vi "NMRvmeCard6.vi"() -> ()   [LabVIEW 2013]
uses:
  <vilib>/Utility/file.llb/Read From Spreadsheet File (DBL).vi
  <vilib>/Analysis/NI_AALBase.lvlib
panel:
  out "Diff Sigma":dbl=0.0021417004437574343 format="%#_13g"
  out "Peak center (MHz)":sgl=213.00386 format="%.3f"
  out "Peak width (MHz)":sgl=0.03243152 format="%.5f"
  in  "Max":bool
  in  "Logoffset (V)":dbl=-5.996000000000003 min=-9.0 max=0.0 step=0.0005 format="%_5g"
  in  "Phase (V)":dbl=6.500000000000002 min=0.0 max=9.0 step=0.0005 format="%_5g"
  out "Telnet error out":errorcluster
  in  "Real/Quad Q curve":bool=TRUE
  out "Temperature (C)":dbl(graph)=26.25
  out "+3V supply":dbl=3.245 format="%_4g"
  out "Temp (C)":dbl=26.25 format="%_4g"
  in  "RemovePed":bool=TRUE
  in  "IF / LOG Det":bool
  in  "Q curve file":string="realback212a.txt"
  out "File name 2":string="C:\\users\\plm\\Desktop\\rssmt\\realback212a.txt"
  in  "AutoTune":bool
  out "RF OK":bool=TRUE
  out "Peak area (V-MHz)":sgl=0.0028527237 format="%.5f"
  in  "Gauss Fit":bool
  out "NMR Graph + Fit":cluster{cluster{dbl, "Numeric":dbl}[]}[](graph)=[{[{212.6, "Numeric"=-0.001303666666666866}, {212.60999999999999, "Numeric"=-0.0012636666666681479}, {212.62, "Numeric"=-0.00035966666666543273}, {212.63, "Numeric"=-0.0006916666666666911}, {212.64, "Numeric"=-0.00025966666666788624}, {212.65, "Numeric"=-0.0006636666666653777}, {212.66, "Numeric"=-0.00020366666666654307}, {212.67, "Numeric"=0.00012033333333236022}, {212.68, "Numeric"=-0.0002916666666653491}, {212.69, "Numeric"=0.001060333333333583}, {212.7, "Numeric"=0.0009763333333325762}, {212.71, "Numeric"=0.0011563333333346557}, {212.72, "Numeric"=0.0010003333333336792}, {212.73, "Numeric"=0.0015083333333327717}, {212.74, "Numeric"=0.001480333333331924}, {212.75, "Numeric"=0.0017163333333337534}, {212.76, "Numeric"=0.0018163333333329357}, {212.77, "Numeric"=0.0019803333333321847}, {212.78, "Numeric"=0.0016083333333338007}, {212.79, "Numeric"=0.001300333333333079}, {212.8, "Numeric"=0.0008563333333324215}, {212.81, "Numeric"=0.00037633333333382535}, {212.82, "Numeric"=0.000660333333333196}, {212.82999999999998, "Numeric"=0.0012083333333326321}, {212.84, "Numeric"=0.001520333333333822}, {212.85, "Numeric"=0.001796333333333287}, {212.85999999999999, "Numeric"=0.0017363333333328176}, {212.87, "Numeric"=0.0022403333333337943}, {212.88, "Numeric"=0.0025083333333333537}, {212.89, "Numeric"=0.0023403333333329775}, {212.9, "Numeric"=0.003036333333333742}, {212.91, "Numeric"=0.0030963333333333953}, {212.92, "Numeric"=0.002320333333333113}, {212.93, "Numeric"=0.002808333333333664}, {212.94, "Numeric"=0.005660333333333411}, {212.95, "Numeric"=0.006976333333333223}, {212.96, "Numeric"=0.00985633333333356}, {212.97, "Numeric"=0.019200333333333403}, {212.98, "Numeric"=0.034408333333333305}, {212.99, "Numeric"=0.03538033333333328}, {213.0, "Numeric"=0.02571633333333337}, {213.01, "Numeric"=0.021516333333333366}, {213.02, "Numeric"=0.020180333333333432}, {213.03, "Numeric"=0.015108333333333307}, {213.04, "Numeric"=0.014500333333333401}, {213.05, "Numeric"=0.014356333333333561}, {213.06, "Numeric"=0.012676333333333224}, {213.07, "Numeric"=0.015160333333333411}, {213.08, "Numeric"=0.011308333333333663}, {213.09, "Numeric"=0.006820333333333113}, {213.1, "Numeric"=0.003896333333333395}, {213.11, "Numeric"=0.002636333333333742}, {213.12, "Numeric"=0.0027403333333329786}, {213.13, "Numeric"=0.0011083333333333535}, {213.14000000000001, "Numeric"=4.033333333379463e-05}, {213.15, "Numeric"=-0.0013636666666671828}, {213.16, "Numeric"=0.0001963333333332871}, {213.17000000000002, "Numeric"=0.0005203333333338219}, {213.18, "Numeric"=0.002208333333332632}, {213.19, "Numeric"=0.0014603333333331955}, {213.2, "Numeric"=0.0009763333333338252}, {213.21, "Numeric"=0.00035633333333242104}, {213.22, "Numeric"=-0.0006996666666669211}, {213.23, "Numeric"=-0.0023916666666661986}, {213.24, "Numeric"=-0.0017196666666654085}, {213.25, "Numeric"=-0.0012836666666670646}, {213.26, "Numeric"=-0.0025836666666662466}, {213.27, "Numeric"=-0.002919666666665363}, {213.28, "Numeric"=-0.0018916666666672285}, {213.29, "Numeric"=-0.0006996666666663209}, {213.3, "Numeric"=-0.0006436666666653455}, {213.31, "Numeric"=-0.0012236666666674244}, {213.32, "Numeric"=-0.0005396666666664159}, {213.33, "Numeric"=-9.166666666534859e-05}, {213.34, "Numeric"=-0.0004796666666676396}, {213.35, "Numeric"=-3.6666666665425424e-06}, {213.36, "Numeric"=-0.0009636666666653776}, {213.37, "Numeric"=-0.00025966666666788624}, {213.38, "Numeric"=-0.0004916666666666923}, {213.39000000000001, "Numeric"=0.0004403333333345659}, {213.4, "Numeric"=-0.0008636666666681468}]}]
  in  "Amp of Q curve":dbl=1.8000000000000034 min=0.0 max=29.0 step=0.01 format="%_3f"
  in  "Subtract Q curve":bool=TRUE
  out "Pedestal Offset":dbl(graph)=-0.007420833333333359
  out "Pedestal Difference":dbl(graph)=-0.001148999999999757
  out "# Good Spectra":i32=1
  in  "Quality cuts":bool=TRUE
  out "Pedestal OK":bool=TRUE
  out "Sweep #":i32=70
  out "1st Sweep":bool
  out "ADC volts OK":bool=TRUE
  out "Peak Height Distribution":cluster{"Y":dbl[], "Y":dbl[]}[](graph)=[{"Y"=[0.03253033333333327, 0.03253033333333327, 0.03253033333333327, 0.03253033333333327, 0.03253033333333327, 0.03253033333333327, 0.03253033333333327, 0.03253033333333327, 0.03253033333333327, 0.03253033333333327, 0.03253033333333327, 0.03253033333333327, 0.03253033333333327, 0.03253033333333327, 0.03253033333333327, 0.03253033333333327, 0.03253033333333327, 0.03253033333333327, 0.03253033333333327, 0.03253033333333327, 0.03253033333333327, 0.03253033333333327, 0.03253033333333327, 0.03253033333333327, 0.03253033333333327, 0.03253033333333327, 0.03253033333333327, 0.03253033333333327, 0.03253033333333327, 0.03253033333333327, 0.03253033333333327, 0.03253033333333327, 0.03253033333333327, 0.03253033333333327, 0.03253033333333327, 0.03253033333333327, 0.03253033333333327, 0.03253033333333327, 0.03253033333333327, 0.03253033333333327, 0.03253033333333327, 0.03253033333333327, 0.03253033333333327, 0.03253033333333327, 0.03253033333333327, 0.03253033333333327, 0.03253033333333327, 0.03253033333333327, 0.03253033333333327, 0.03253033333333327, 0.03253033333333327, 0.03253033333333327, 0.03253033333333327, 0.03253033333333327, 0.03253033333333327, 0.03253033333333327, 0.03253033333333327, 0.03253033333333327, 0.03253033333333327, 0.03253033333333327, 0.03253033333333327, 0.03253033333333327, 0.03253033333333327, 0.03253033333333327, 0.03253033333333327, 0.03253033333333327, 0.03253033333333327, 0.03253033333333327, 0.03253033333333327, 0.03253033333333327, 0.03253033333333327, 0.03253033333333327, 0.03253033333333327, 0.03253033333333327, 0.03253033333333327, 0.03253033333333327, 0.03253033333333327, 0.03253033333333327, 0.03253033333333327, 0.03253033333333327, 0.03253033333333327, 0.03253033333333327, 0.03253033333333327, 0.03253033333333327, 0.03253033333333327, 0.03253033333333327, 0.03253033333333327, 0.03253033333333327, 0.03253033333333327, 0.03253033333333327, 0.03253033333333327, 0.03253033333333327, 0.03253033333333327, 0.03253033333333327, 0.03253033333333327, 0.03253033333333327, 0.03253033333333327, 0.03253033333333327, 0.03253033333333327, 0.03253033333333327], "Y"=[0.0, 0.0, 0.0, 0.0, 0.0, 0.0, 0.0, 0.0, 0.0, 0.0, 0.0, 0.0, 0.0, 0.0, 0.0, 0.0, 0.0, 0.0, 0.0, 0.0, 0.0, 0.0, 0.0, 0.0, 0.0, 0.0, 0.0, 0.0, 0.0, 0.0, 0.0, 0.0, 0.0, 0.0, 0.0, 0.0, 0.0, 0.0, 0.0, 0.0, 0.0, 0.0, 0.0, 0.0, 0.0, 0.0, 0.0, 0.0, 0.0, 0.0, 0.0, 0.0, 0.0, 0.0, 0.0, 0.0, 0.0, 0.0, 0.0, 0.0, 0.0, 0.0, 0.0, 0.0, 0.0, 0.0, 0.0, 0.0, 0.0, 0.0, 0.0, 0.0, 0.0, 0.0, 0.0, 0.0, 0.0, 0.0, 0.0, 0.0, 0.0, 0.0, 0.0, 0.0, 0.0, 0.0, 0.0, 0.0, 0.0, 0.0, 0.0, 0.0, 0.0, 0.0, 0.0, 0.0, 0.0, 0.0, 0.0, 1.0]}]
  in  "# of Sweeps":i32=1000
  out "S/N":dbl=nan format="%_3g"
  out "Peak mean (V)":dbl=0.03253033333333327 format="%_4g"
  out "Peak Height":dbl(graph)=0.03538033333333328
  in  "Raw Data":bool=TRUE
  in  "Tank RF":bool=TRUE
  in  "IF Atten (dB)":i8=3 min=0 max=31 step=1
  in  "IFoffset (V)":dbl=5.366811000000014 min=-0.0 max=9.0 step=0.001 format="%.4f"
  in  "Tune  (V)":dbl=0.34700000000000086 min=-0.5 max=8.0 step=0.001 format="%.4f"
  in  "Hi / Lo Gain":bool
  out "Voltage Array":sgl[](array[numeric])=[0.0208, 0.0194, 0.0189, 0.0172, 0.0163, 0.0146, 0.0138, 0.0129, 0.0113, 0.0115, 0.0103, 0.0094, 0.0082, 0.0077, 0.0067, 0.006, 0.0052, 0.0045, 0.0033, 0.0022, 0.001, -0.0002, -0.0006, -0.0007, -0.001, -0.0013, -0.0019, -0.0019, -0.0021, -0.0027, -0.0024, -0.0027, -0.0038, -0.0036, -0.001, 0.0001, 0.0028, 0.012, 0.0271, 0.028, 0.0183, 0.0141, 0.0128, 0.0078, 0.0073, 0.0073, 0.0058, 0.0085, 0.0049, 0.0007, -0.0019, -0.0028, -0.0023, -0.0035, -0.0041, -0.005, -0.0029, -0.002, 0.0003, 0.0002, 0.0004, 0.0005, 0.0002, -0.0007, 0.0008, 0.0021, 0.0017, 0.0023, 0.0043, 0.0065, 0.0076, 0.0081, 0.0099, 0.0115, 0.0123, 0.014, 0.0143, 0.0163, 0.0174, 0.0197, 0.0198] format="%.4f"
  in  "Invert Polarity":bool=TRUE
  out "Pedestal Diff (V)":sgl=-0.001149 format="%.3f"
  out "Peak amp (V)":sgl=0.035380334 format="%.3f"
  in  "Save Data to File":bool
  in  "RF Level (dBm)":dbl min=-10.0 max=10.0 step=0.1 format="%.2f"
  out "SMT error out":errorcluster
  out "Sample RMS (V)":dbl=0.0007950617283950617 format="%.4f"
  in  "# Sample/step":i32=70 min=1 max=5000 step=100
  in  "Step Width (MHz)":dbl=0.01 min=0.0 max=1000.0 step=0.0001 format="%.4f"
  in  "Freq Span (MHz)":dbl=0.8 min=0.0 max=3000.0 step=0.1 format="%.3f"
  in  "Center Freq (MHz)":dbl=213.0 min=0.005 max=6000.0 step=0.1 format="%.3f"
  in  "Sweep Mode":u16(ring)=3 items=["Off", "Single", "Auto", "Step"]
  in  "GPIB Addr (28)":refnum<visa-resource-name>="GPIB0::28::INSTR"
  # "E1039 Prototype NMR Control Panel"
  # "Settings"
  # "D\nA\nC"
  # "R\nF\n\nG\nE\nN \n\n+\n\nI\nF"
  # "A\nD\nC"
  # "I\n/\nO"
  # "D\nA\nT\nA\n\nA \nN\nA\nL\nY\nS\nI\nS"
  # "Results"
  # "A\nv\ne\nr\na\ng\ne"
  # "S\nw\ne\ne\np"
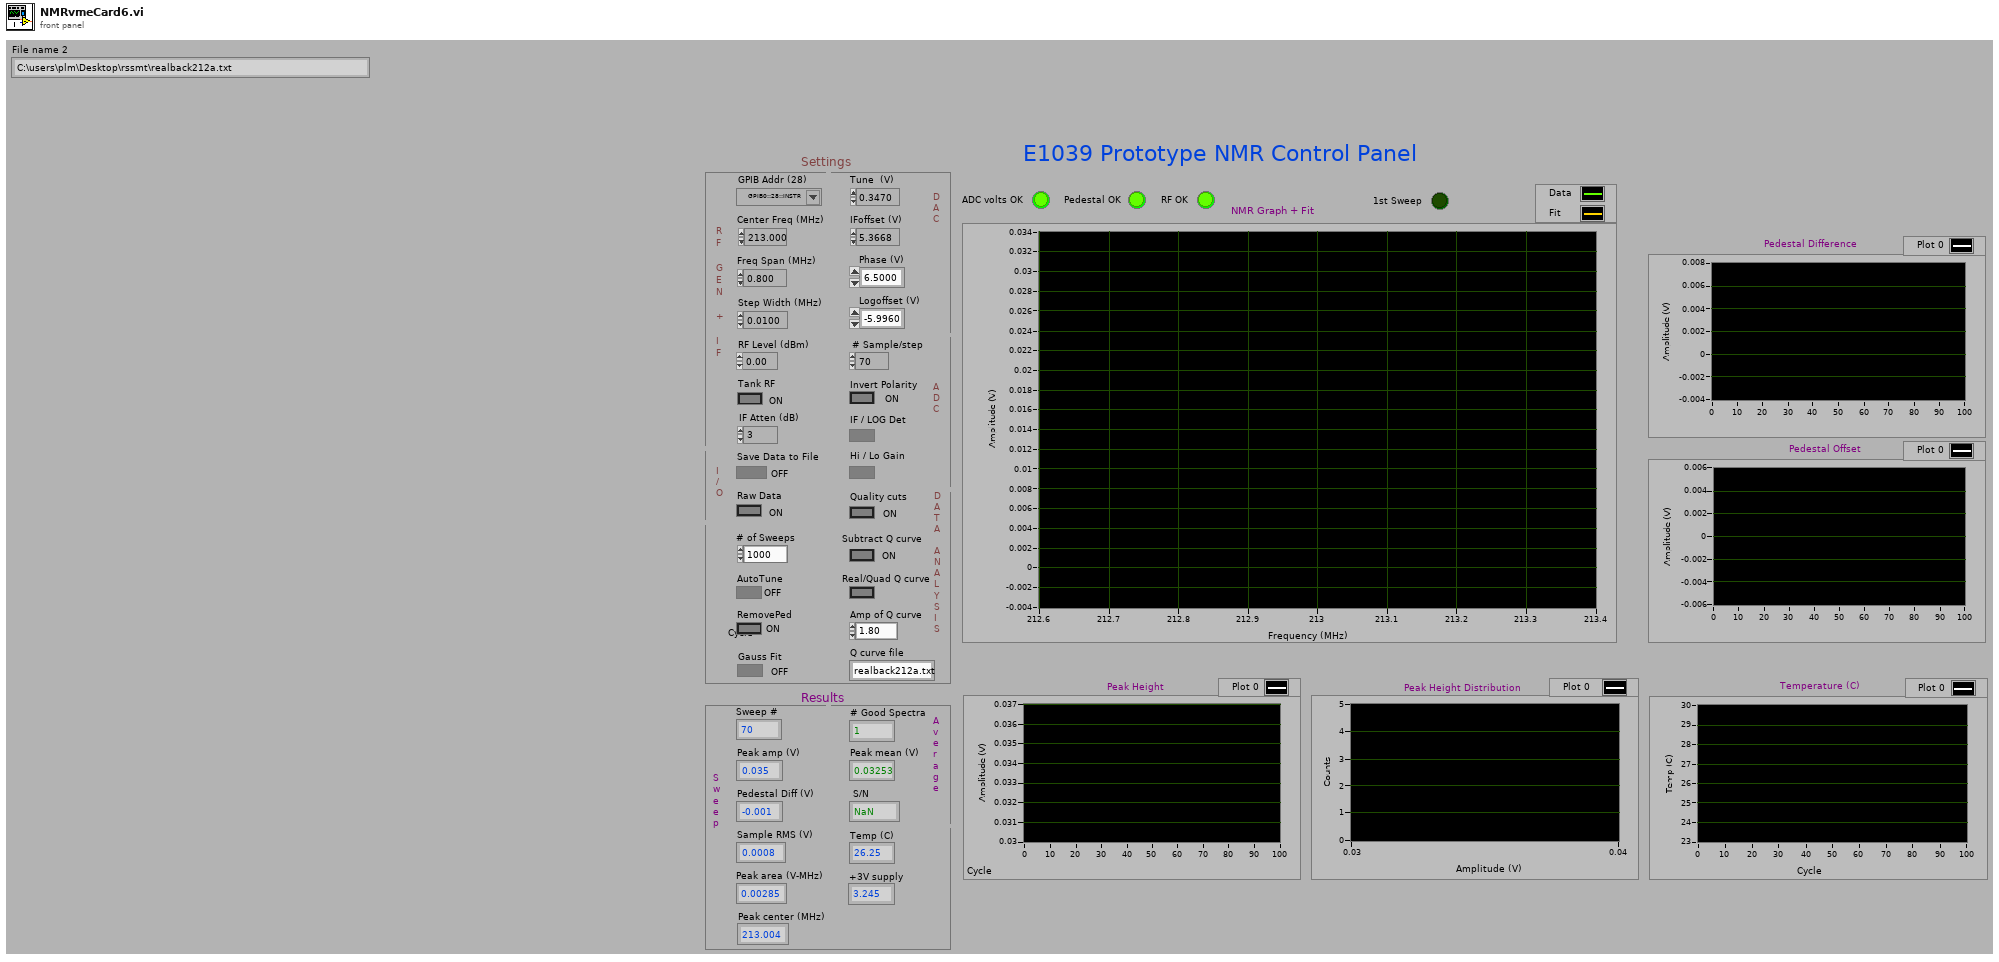
[diagram p1: front panel]
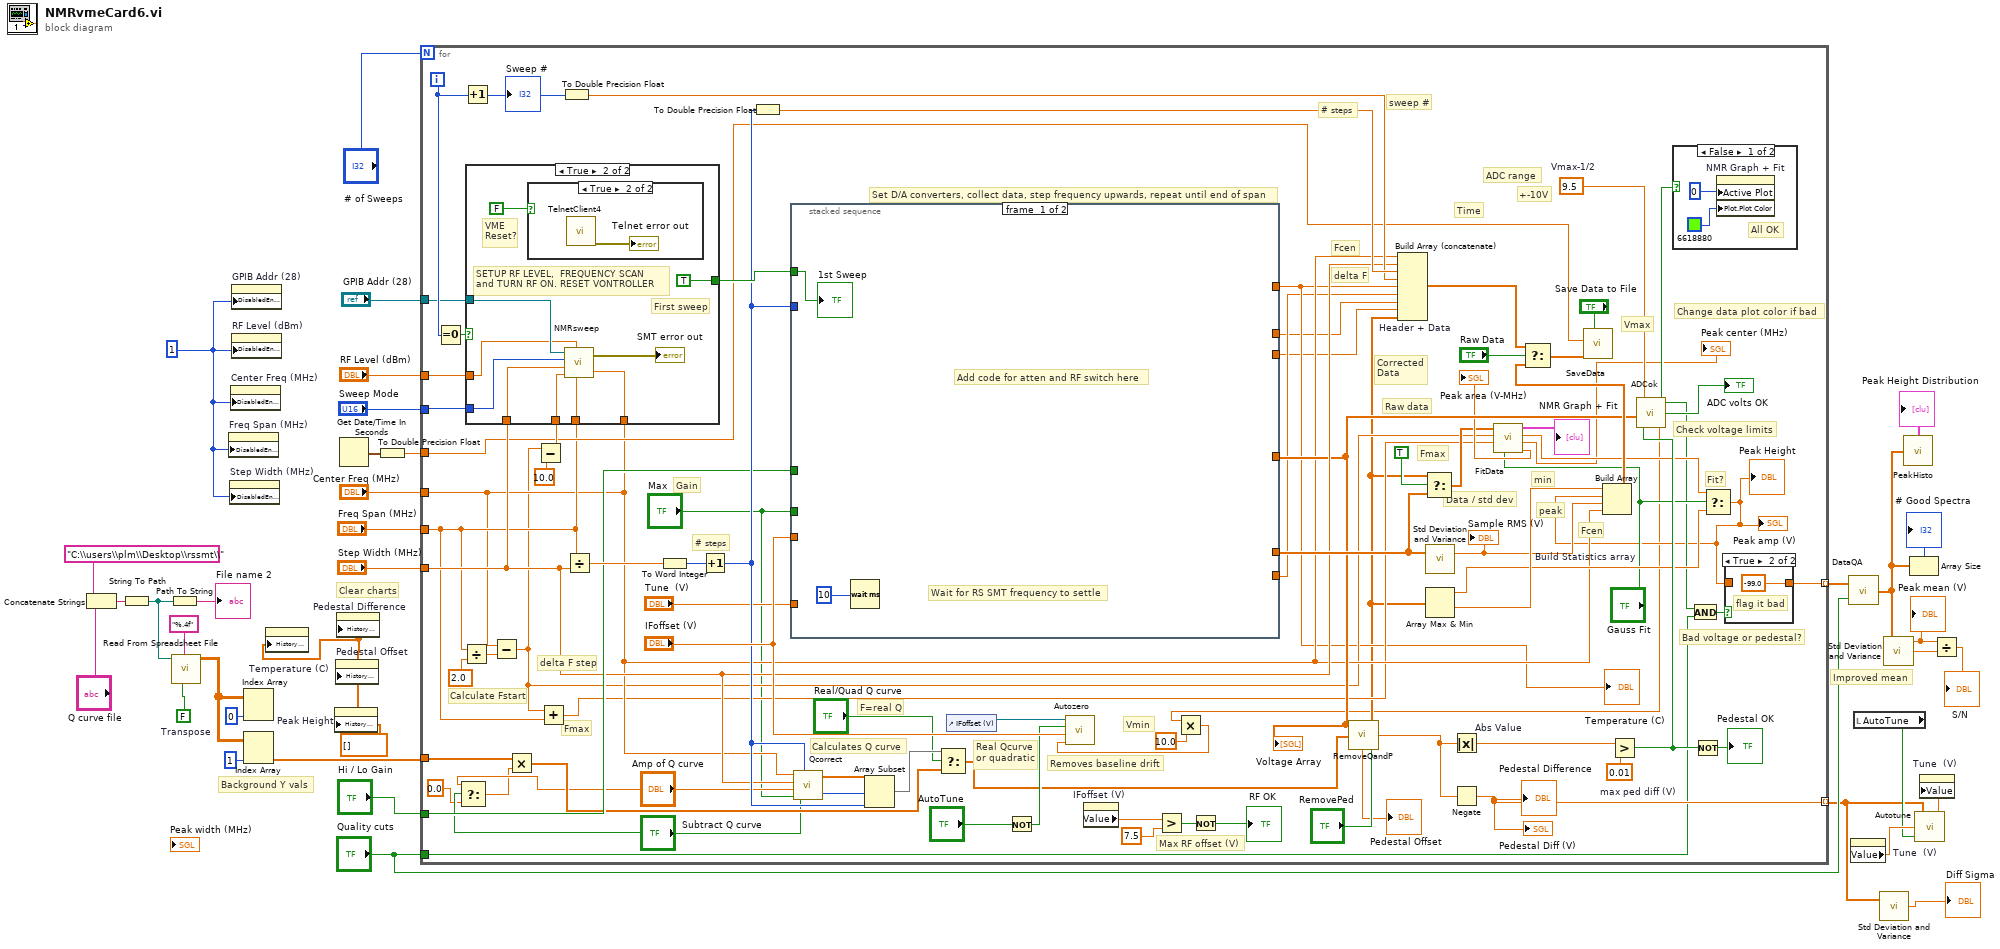
[diagram p0: block diagram]
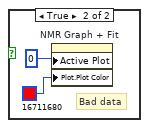
[diagram p2: hidden frame]
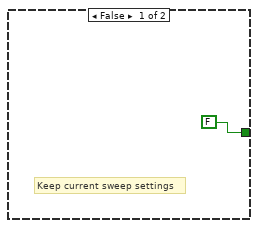
[diagram p4: hidden frame]
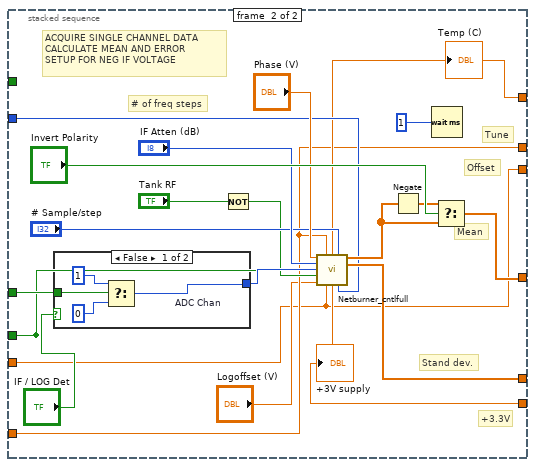
[diagram p6: hidden frame]
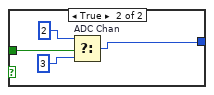
[diagram p7: hidden frame]
diagram:
  w4 = 1
  w16 = FALSE  # Transpose
  w8 = dbl[] []
  # "Background Y vals"
  # "Clear charts"
  # "Improved mean"
  n1 = Concatenate Strings "Concatenate Strings"("C:\\users\\plm\\Desktop\\rssmt\\", "Q curve file") -> (w19:string)
  n2 = String To Path(string=w19) -> (path=w15:path)
  n3 = Path To String(path=w15) -> (string=→"File name 2":string)
  n4 = call-poly <vilib>:"Read From Spreadsheet File.vi"("transpose (no:F)"=w16, "format (%.3f)"="%.4f", "file path (dialog if empty)"=w15) -> ("all rows"=w14:dbl[][])  [unwired: 4 in, 4 out]
  n5 = property on="Freq Span (MHz)" class="DigNum (strict)"("DisabledEnum"=w4) -> ()  [unwired: 2 in, 2 out]
  n6 = property on="Step Width (MHz)" class="DigNum (strict)"("DisabledEnum"=w4) -> ()  [unwired: 2 in, 2 out]
  n7 = property on="Center Freq (MHz)" class="DigNum (strict)"("DisabledEnum"=w4) -> ()  [unwired: 2 in, 2 out]
  n8 = property on="GPIB Addr (28)" class="VISAName"("DisabledEnum"=w4) -> ()  [unwired: 2 in, 2 out]
  n9 = property on="RF Level (dBm)" class="DigNum (strict)"("DisabledEnum"=w4) -> ()  [unwired: 2 in, 2 out]
  n10 = Index Array "Index Array"(array=w14, index (col)=0) -> ()  [unwired: 1 in, 1 out]
  n11 = Index Array(array=w14, index (col)=1) -> (element=w9:dbl[])  [unwired: 1 in]
  n12 = property on="Temperature (C)" class="WFChart (strict)"("History Data"=w8) -> ()  [unwired: 2 in, 2 out]
  n13 = property on="Peak Height" class="WFChart (strict)"("History Data"=w8) -> ()  [unwired: 2 in, 2 out]
  n14 = property on="Pedestal Offset" class="WFChart (strict)"("History Data"=w8) -> ()  [unwired: 2 in, 2 out]
  n15 = property on="Pedestal Difference" class="WFChart (strict)"("History Data"=w8) -> ()  [unwired: 2 in, 2 out]
  n16 = Get Date/Time In Seconds() -> (seconds since 1Jan1904=w21:timestamp)
  n17 = To Double Precision Float(number=w21) -> (double precision float=w20:dbl)
  n18 = for {
    N: "# of Sweeps" -> [_]
    tunnel: [w104] -> w34 mode=indexing
    tunnel: "Quality cuts" -> [w83]
    tunnel: [w88] -> w2 mode=indexing
    tunnel: "Center Freq (MHz)" -> [w70]
    tunnel: "Freq Span (MHz)" -> [w76]
    tunnel: "Step Width (MHz)" -> [w82]
    tunnel: "Sweep Mode" -> [w92]
    tunnel: "Hi / Lo Gain" -> [w91]
    tunnel: "GPIB Addr (28)" -> [w90]
    tunnel: "RF Level (dBm)" -> [w89]
    tunnel: w20 -> [w77]
    tunnel: w9 -> [w55]
    i -> [w102]
    w86 = 9.5  # Vmax-1/2
    w105 = 0.01  # max ped diff (V)
    # "Gain"
    # "F=real Q"
    # "Real Qcurve\nor quadratic"
    # "+-10V"
    # "Vmax"
    # "Change data plot color if bad"
    # "Max RF offset (V)"
    # "Fmax"
    # "Fit?"
    # "Fmax"
    # "Time"
    # "Vmin"
    # "min"
    # "peak"
    # "Raw data"
    # "Corrected\nData"
    # "Fcen"
    # "delta F"
    # "# steps"
    # "ADC range"
    # "sweep #"
    # "Fcen"
    # "Set D/A converters, collect data, step frequency upwards, repeat until end of span"
    # "Calculates Q curve"
    # "Removes baseline drift"
    # "Bad voltage or pedestal?"
    # "Check voltage limits"
    # "Data / std dev"
    # "# steps"
    # "Calculate Fstart"
    # "delta F step"
    n19 = Equal To 0?(x=w102) -> (x = 0?=w107:bool)
    n20 = Select(t="Amp of Q curve", s="Subtract Q curve", f=0.0) -> (s? t:f=w50:dbl)
    n21 = Divide(x=w76, y=sgl 2.0) -> (x/y=w118:dbl)
    n22 = Increment(x=w102) -> (x+1=w93:i32)
    "Sweep #" <- w93
    n23 = Subtract(x=w70, y=w118) -> (x-y=w65:dbl)
    n24 = Multiply(x=w55, y=w50) -> (x*y=w54:dbl[])
    n25 = Subtract(x=w65, y=10.0) -> (x-y=w116:dbl)
    n26 = case shown="True" w107 {
      tunnel: w116 -> [_ w137]
      tunnel: w82 -> [_ w135]
      tunnel: w70 -> [_ w134]
      tunnel: w76 -> [_ w136]
      tunnel: [FALSE TRUE] -> w106
      tunnel: w92 -> [_ w131]
      tunnel: w90 -> [_ w130]
      tunnel: w89 -> [_ w129]
      frame False {
        # "Keep current sweep settings"
      }
      frame True {
        # "VME\nReset?"
        # "First sweep"
        # "SETUP RF LEVEL,  FREQUENCY SCAN\nand TURN RF ON. RESET VONTROLLER"
        n27 = case shown="True" FALSE {
          frame False {
          }
          frame True {
            n28 = call "TelnetClient4.vi"() -> ("Telnet error"=→"Telnet error out":errorcluster)  [unwired: 4 in, 3 out]
          }
        }
        n29 = call "NMRsweep.vi"("Center Freq (MHz)"=w134, "Freq Span (MHz)"=w136, "RF Level (dBm)"=w129, "Foffset (MHz)"=w137, "Step Width (MHz)"=w135, "Sweep Mode"=w131, "GPIB Addr (28)"=w130) -> ("error out"=→"SMT error out":errorcluster)
      }
    }
    n30 = Add(x=w65, y=w76) -> (x+y=w64:dbl)
    n31 = To Double Precision Float(number=w93) -> (double precision float=w94:dbl)
    n32 = Divide(x=w76, y=w82) -> (x/y=w120:dbl)
    n33 = To Word Integer(number=w120) -> (16bit integer=w117:i16)
    n34 = Increment(x=w117) -> (x+1=w96:i16)
    n35 = To Double Precision Float(number=w96) -> (double precision float=w95:dbl)
    n36 = stacked-sequence {
      tunnel: [_ w152] -> w110
      tunnel: [_ w159] -> w80
      tunnel: w96 -> [_ w149]
      tunnel: "IFoffset (V)" -> [_ w142]
      tunnel: w91 -> [_ w157]
      tunnel: w106 -> [w139 _]
      tunnel: "Tune  (V)" -> [_ w144]
      tunnel: [_ w148] -> w46
      tunnel: [_ w145] -> w45
      tunnel: [_ w144] -> w43
      tunnel: [_ w142] -> w42
      tunnel: [_ w141] -> _
      tunnel: "Max" -> [_ w141]
      frame #0 {
        # "Add code for atten and RF switch here"
        # "Wait for RS SMT frequency to settle"
        n37 = Wait (ms)(milliseconds to wait=10) -> ()  [unwired: 1 out]
        "1st Sweep" <- w139
      }
      frame #1 {
        # "+3.3V"
        # "Offset"
        # "Tune"
        # "Stand dev."
        # "Mean"
        # "ACQUIRE SINGLE CHANNEL DATA\nCALCULATE MEAN AND ERROR\nSETUP FOR NEG IF VOLTAGE"
        # "# of freq steps"
        n38 = case shown="False" "IF / LOG Det" {
          tunnel: w157 -> [w165 w166]
          tunnel: [w162 w167] -> w151
          frame False {
            n39 = Select "ADC Chan"(t=1, s=w165, f=0) -> (s? t:f=w162:i32)
          }
          frame True {
            n40 = Select "ADC Chan"(t=2, s=w166, f=3) -> (s? t:f=w167:i32)
          }
        }
        n41 = Not(x="Tank RF") -> (.not. x?=w147:bool)
        n42 = call "Netburner_cntlfull.vi"("Phase Volt"="Phase (V)", "Tune Volt"=w144, "# Data"="# Sample/step", "IF Atten (dB)"="IF Atten (dB)", "NMR ADC"=w151, "Hi Gain"=w141, "Tank RF"=w147, "LogOff Volt"="Logoffset (V)", "IFOff Volt"=w142, "# f steps"=w149) -> ("Temp (C)"=w148:dbl, "ADC value"=w153:dbl[], "ADC error"=w152:dbl[], "Volts"=w145:dbl)  [unwired: 2 out]
        "Temp (C)" <- w148
        "+3V supply" <- w145
        n43 = Negate(x=w153) -> (-x=w158:dbl[])
        n44 = Wait (ms)(milliseconds to wait=1) -> ()  [unwired: 1 out]
        n45 = Select(t=w158, s="Invert Polarity", f=w153) -> (s? t:f=w159:dbl[])
      }
    }
    "Voltage Array" <- w80
    "Temperature (C)" <- w46
    n46 = call "Qcorrect.vi"("Subtract Q curve"="Subtract Q curve", "Nstep"=w96, "Max Gain"="Max", "Amp of Q curve"="Amp of Q curve", "Step Width (MHz)"=w82, "Center Freq (MHz)"=w70) -> ("Start"=w111:i32, "Array"=w112:dbl[])
    n47 = Array Subset "Array Subset"(array=w112, index=w111, length=w96) -> (w58:dbl[])
    n48 = Select(t=w58, s="Real/Quad Q curve", f=w54) -> (s? t:f=w57:dbl[])
    n49 = control-ref of="IFoffset (V)"() -> (w85:refnum<vi>)
    n50 = Not(x="AutoTune") -> (.not. x?=w59:bool)
    n51 = property on="IFoffset (V)" class="DigNum (strict)"() -> ("Value"=w74:dbl)  [unwired: 2 in, 2 out]
    n52 = Greater?(x=w74, y=7.5) -> (0:w72:bool)
    n53 = Not(x=w72) -> (.not. x?=→"RF OK":bool)
    n54 = call "RemoveQandP.vi"("Subtract Ped?"="RemovePed", "Qcurve"=w57, "Raw data"=w80) -> ("Ped L-R"=w98:dbl, "Corrected data"=w44:dbl[], "Ped Offfset"=→"Pedestal Offset":dbl)
    n55 = Build Array (concatenate) "Header + Data"(w70, w82, w95, w94, w46, w45, w43, w42, w44) -> (w97:dbl[])
    n56 = Select(t=w44, s=TRUE, f=w110) -> (s? t:f=w66:dbl[])
    n57 = call <vilib>:"Std Deviation and Variance.vi"("X"=w110) -> ("mean"=w81:dbl)  [unwired: 1 in, 2 out]
    "Sample RMS (V)" <- w81
    n58 = Array Max & Min(array=w44) -> (max value=w75:dbl, min value=w109:dbl)  [unwired: 2 out]
    n59 = Absolute Value "Abs Value"(x=w98) -> (abs(x)=w100:dbl)
    n60 = Negate(x=w98) -> (-x=w88:dbl)
    "Pedestal Diff (V)" <- w88
    "Pedestal Difference" <- w88
    n61 = call "FitData.vi"("Fit?"="Gauss Fit", "Fmax"=w64, "Fmin"=w65, "Yarray"=w66) -> ("Peak Area (V-MHz)"=→"Peak area (V-MHz)":dbl, "Center Freq (MHz)"=→"Peak center (MHz)":dbl, "Amplitude (V)"=w68:dbl, "NMR Graph + Fit"=→"NMR Graph + Fit":cluster{cluster{dbl, "Numeric":dbl}[]}[])  [unwired: 1 out]
    n62 = Greater?(x=w100, y=w105) -> (0:w87:bool)
    n63 = call "ADCok.vi"("PedOK"=w87, "Array"=w80, "Vmax-1/2"=w86) -> ("Vmin"=w39:dbl, "ADC voltages OK"=→"ADC volts OK":bool, "Allok"=w62:bool)
    n64 = Multiply(x=w39, y=10.0) -> (x*y=w37:dbl)
    n65 = call "Autozero.vi"("Vmin (V)"=w37, "IFoffset (V)"="IFoffset (V)", "Enable"=w59, "reference"=w85) -> ()
    n66 = case shown="False" w62 {
      frame False {
        # "All OK"
        n67 = property on="NMR Graph + Fit" class="XYGraph (strict)"("Active Plot"=0, "Plot.Plot Color"=u32 6618880) -> ()  [unwired: 2 in, 2 out]
      }
      frame True {
        # "Bad data"
        n68 = property on="NMR Graph + Fit" class="XYGraph (strict)"("Active Plot"=0, "Plot.Plot Color"=u32 16711680) -> ()  [unwired: 2 in, 2 out]
      }
    }
    n69 = And(x=w62, y=w83) -> (x .and. y?=w101:bool)
    n70 = Not(x=w87) -> (.not. x?=→"Pedestal OK":bool)
    n71 = Select(t=w68, s="Gauss Fit", f=w75) -> (s? t:f=w61:dbl)
    "Peak amp (V)" <- w61
    "Peak Height" <- w61
    n72 = Build Array "Build Statistics array"(w109, w61, w81, w70) -> (w115:dbl[])
    n73 = Select(t=w97, s="Raw Data", f=w115) -> (s? t:f=w78:dbl[])
    n74 = call "SaveData.vi"("Array"=w78, "Save Data to File"="Save Data to File", "Ext time (sec)"=w77) -> ()  [unwired: 1 out]
    n75 = case shown="True" w101 {
      tunnel: [w125 -99.0] -> w104
      tunnel: w61 -> [w125 _]
      frame False {
        # "Data OK"
      }
      frame True {
        # "flag it bad"
      }
    }
  }
  n76 = call "DataQA.vi"("Quality cuts"="Quality cuts", "Data In"=w34) -> ("Data Out"=w33:dbl[])
  n77 = property on="Tune  (V)" class="DigNum (strict)"() -> ("Value"=w24:dbl)  [unwired: 2 in, 2 out]
  n78 = local read "AutoTune"() -> (w3:bool)
  n79 = call <vilib>:"Std Deviation and Variance.vi"("X"=w2) -> ("standard deviation"=→"Diff Sigma":dbl)  [unwired: 1 in, 2 out]
  n80 = call <vilib>:"Std Deviation and Variance.vi"("X"=w33) -> ("mean"=w7:dbl, "standard deviation"=w6:dbl)  [unwired: 1 in, 1 out]
  "Peak mean (V)" <- w7
  n81 = call "PeakHisto.vi"("Data Out"=w33) -> ("XY Graph"=→"Peak Height Distribution":cluster{"Y":dbl[], "Y":dbl[]}[])
  n82 = Array Size(array=w33) -> (size(s)=→"# Good Spectra":i32)
  n83 = call "Autotune.vi"("Adjust Tune"=w3, "Tune Vin"=w24, "Pedestal Diff"=w2) -> ("Tune Vout"=w23:dbl)
  n84 = property on="Tune  (V)" class="DigNum (strict)"("Value"=w23) -> ()  [unwired: 2 in, 2 out]
  n85 = Divide(x=w7, y=w6) -> (x/y=→"S/N":dbl)
